vi "Get Config.vi"(8 "error in (no error)":errorcluster, 11 "DeploySerialResource in":refnum<class "SerialResource.lvclass">) -> (0 "error out":errorcluster, 2 "Config":T1[](array[typedef]), 3 "DeploySerialResource out":refnum<class "SerialResource.lvclass">)   [LabVIEW 2020, in "PicoG-Core.lvlib" / "SerialResource.lvclass"]
uses:
  SerialResource.lvclass
  SerialResource.lvclass/SerialResource.ctl
  Resource/Config Item.ctl
  Resource/Resource.lvclass
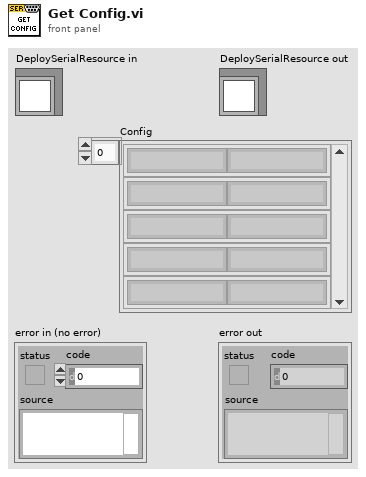
[diagram p1: front panel]
types:
  T1 = typedef "PicoG-Core.lvlib/Resource.lvclass/Config Item.ctl" = cluster{"Key":string, "Value":string}
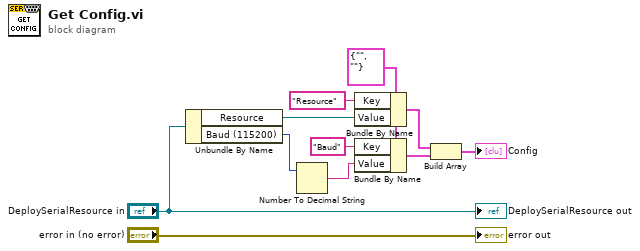
[diagram p0: block diagram]
diagram:
  w9 = T1 {"Key"="", "Value"=""} ("Config Item")
  n1 = Unbundle By Name("DeploySerialResource in") -> ("Resource"=w8:refnum<visa-resource-name>, "Baud (115200)"=w10:u32)
  n2 = Number To Decimal String(number=w10) -> (decimal integer string=w5:string)  [unwired: 1 in]
  n3 = Bundle By Name(cluster=w9, "Key"="Resource", "Value"=w8) -> (w4:T1)
  n4 = Bundle By Name(cluster=w9, "Key"="Baud", "Value"=w5) -> (w3:T1)
  n5 = Build Array(w4, w3) -> (→"Config":T1[])
  "error out" <- "error in (no error)"
  "DeploySerialResource out" <- "DeploySerialResource in"
